vi "add_function.vi"(8 "error in":errorcluster, 9 "BD Position":cluster{"Left":i32, "Top":i32}, 10 "Function Type":i32, 11 "VI Ref In":refnum<vi>) -> (0 "error out":errorcluster, 2 "Node Refnum":refnum<vi>, 3 "VI Ref Out":refnum<vi>)   [LabVIEW 2018]
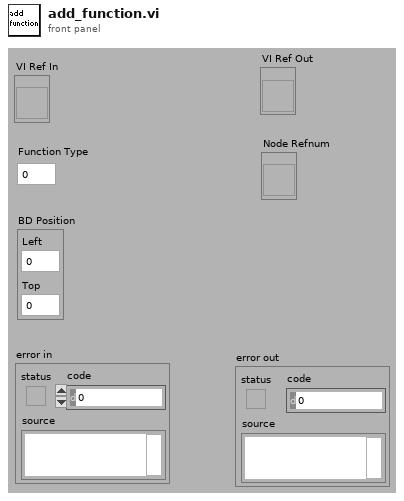
[diagram p1: front panel]
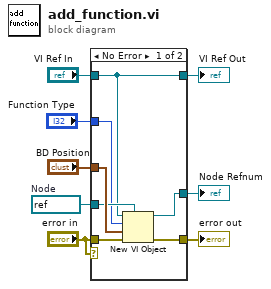
[diagram p0: block diagram]
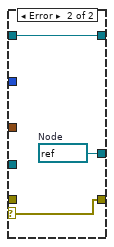
[diagram p2: hidden frame]
diagram:
  w4 = refnum<vi> refnum  # Node
  n1 = case shown="No Error" "error in" {
    selector: "error in" -> [_ w18]
    tunnel: "error in" -> [w15 _]
    tunnel: "VI Ref In" -> [w10 w16]
    tunnel: [w9 w18] -> w7
    tunnel: [w14 w17] -> w6
    tunnel: "BD Position" -> [w13 _]
    tunnel: w4 -> [w12 _]
    tunnel: "Function Type" -> [w11 _]
    tunnel: [w10 w16] -> w1
    frame No Error {
      n2 = New VI Object(vi object class=w12, owner refnum=w10, style=w11, position/next to=w13, 8:w15) -> (object refnum=w14:refnum<vi>, 0:w9:errorcluster)  [unwired: 3 out]
    }
    frame Error {
      w17 = refnum<vi> refnum  # Node
    }
  }
  "error out" <- w7
  "Node Refnum" <- w6
  "VI Ref Out" <- w1
